vi "Control LV PowerSupply.vi"(8 "error in":errorcluster, 9 "Socket Index":i16, 11 "PPS Config In":T1={"VISA Resource"="", "Voltage Level (0.0 V)"=0.0, "CURRent Limit (0.0 A)"=0.0, "OVP LEVEL (0V)"=0.0, "Enable OVP (T: Enable)"=TRUE, "OCP LEVEL (0A)"=0.0, "Enable OCP (T: Enable)"=TRUE, "Value Out"="", "Value In"="", "Actual Voltage Level (V)"=0.0, "Actual Current Limit (A)"=0.0, "Select Instrument"="", "Enable Output"=FALSE, "PPS Operation"=enum."Close", "Type"=0} {"Type" items=["Voltage", "Current"]; "Actual Current Limit (A)" format="%.2f"; "Actual Voltage Level (V)" format="%.2f"; "OCP LEVEL (0A)" format="%.2f"; "OVP LEVEL (0V)" format="%.2f"; "Voltage Level (0.0 V)" format="%.2f"}) -> (0 "error out":errorcluster, 2 "Report Text":string, 3 "PPS Config Out":T1={"VISA Resource"="", "Voltage Level (0.0 V)"=0.0, "CURRent Limit (0.0 A)"=0.0, "OVP LEVEL (0V)"=0.0, "Enable OVP (T: Enable)"=TRUE, "OCP LEVEL (0A)"=0.0, "Enable OCP (T: Enable)"=TRUE, "Value Out"="", "Value In"="", "Actual Voltage Level (V)"=0.0, "Actual Current Limit (A)"=0.0, "Select Instrument"="", "Enable Output"=FALSE, "PPS Operation"=enum."Close", "Type"=0} {"Type" items=["Voltage", "Current"]; "Actual Current Limit (A)" format="%.2f"; "Actual Voltage Level (V)" format="%.2f"; "OCP LEVEL (0A)" format="%.2f"; "OVP LEVEL (0V)" format="%.2f"; "Voltage Level (0.0 V)" format="%.2f"})   [LabVIEW 2023, in "HardwareAbstractionLayer_LVOOP.lvlib" / "Wait Monitor.lvclass"]
uses:
  Wait Monitor.lvclass
  PowerSupply/Teststand/Control/PPS StepType Control.ctl
  PowerSupply/IT-M3904D/IT-M3904D.lvclass
  PowerSupply/Control/PPS Configure Data.ctl
  PowerSupply/PowerSupply.lvclass
  Database/Database.lvclass
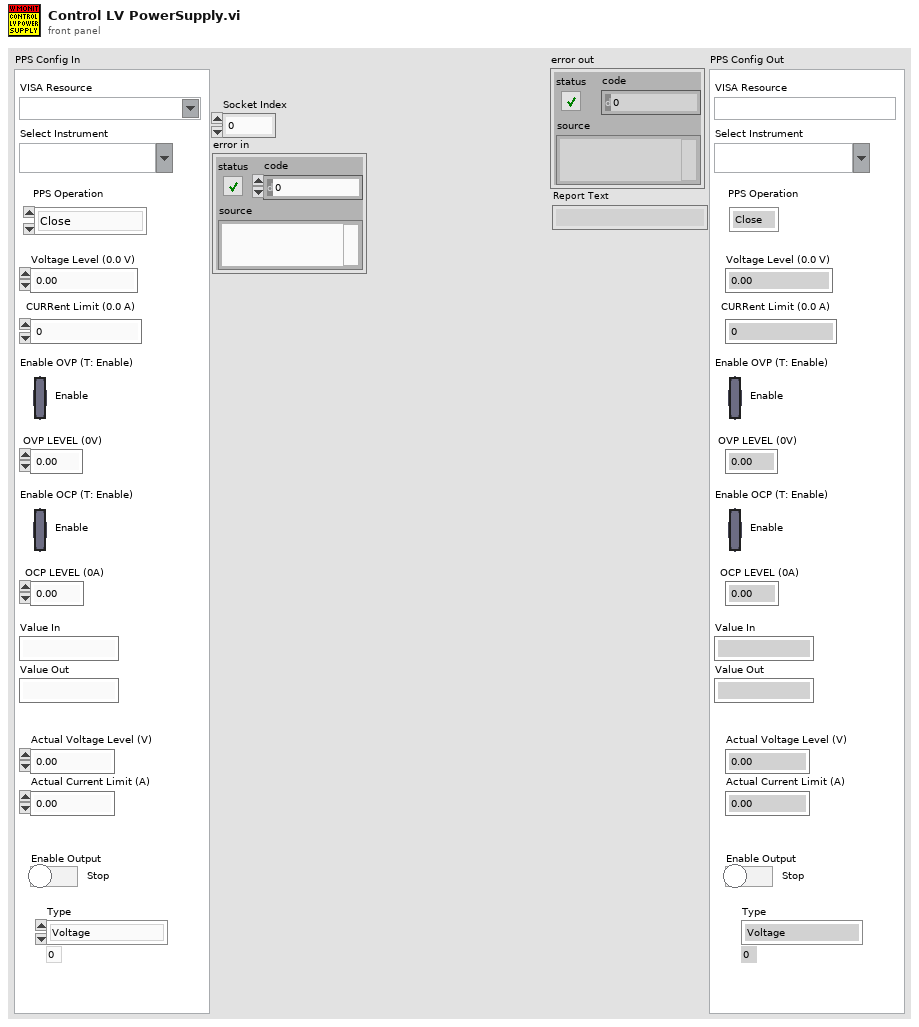
[diagram p1: front panel]
types:
  T1 = typedef "HardwareAbstractionLayer_LVOOP.lvlib/PowerSupply.lvclass/PPS StepType Control.ctl" = cluster{"VISA Resource":refnum<visa-resource-name>, "Voltage Level (0.0 V)":dbl, "CURRent Limit (0.0 A)":dbl, "OVP LEVEL (0V)":dbl, "Enable OVP (T: Enable)":bool, "OCP LEVEL (0A)":dbl, "Enable OCP (T: Enable)":bool, "Value Out":string, "Value In":string, "Actual Voltage Level (V)":dbl, "Actual Current Limit (A)":dbl, "Select Instrument":string, "Enable Output":bool, "PPS Operation":enum32{"Init", "Self Test", "Configure", "Measure", "Close"}, "Type":u16}
  T2 = typedef "HardwareAbstractionLayer_LVOOP.lvlib/PowerSupply.lvclass/PPS Configure Data.ctl" = cluster{"Voltage Level (0.0 V)":dbl, "CURRent Limit (0.0 A)":dbl, "OVP LEVEL (0V)":dbl, "OCP LEVEL (0A)":dbl, "Enable OVP (T: Enable)":bool, "Enable OCP (T: Enable)":bool, "Enable Output ":bool, "Delays OCP":dbl, "Delays OVP":dbl, "Mode(0:Voltage)":u16, "CURRent Level (0.0 A)":dbl, "Voltage Limit (0.0 V)":dbl}
  T3 = enum32{"Init", "Self Test", "Configure", "Measure", "Close"}
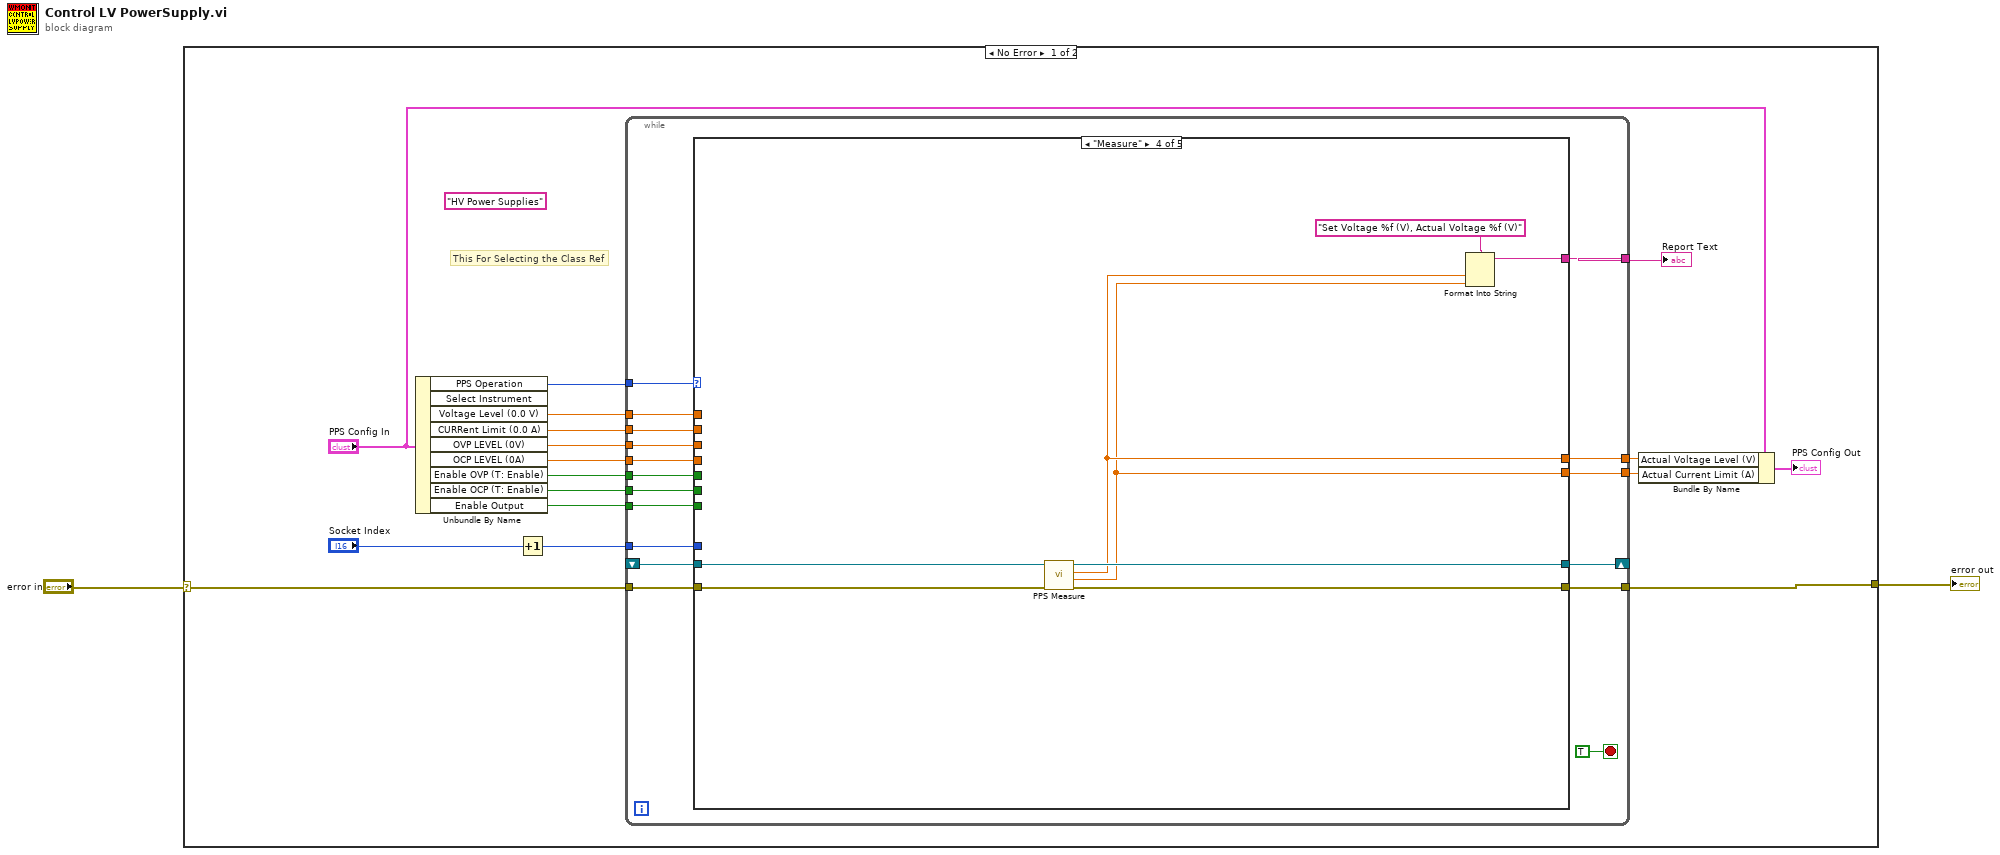
[diagram p0: block diagram]
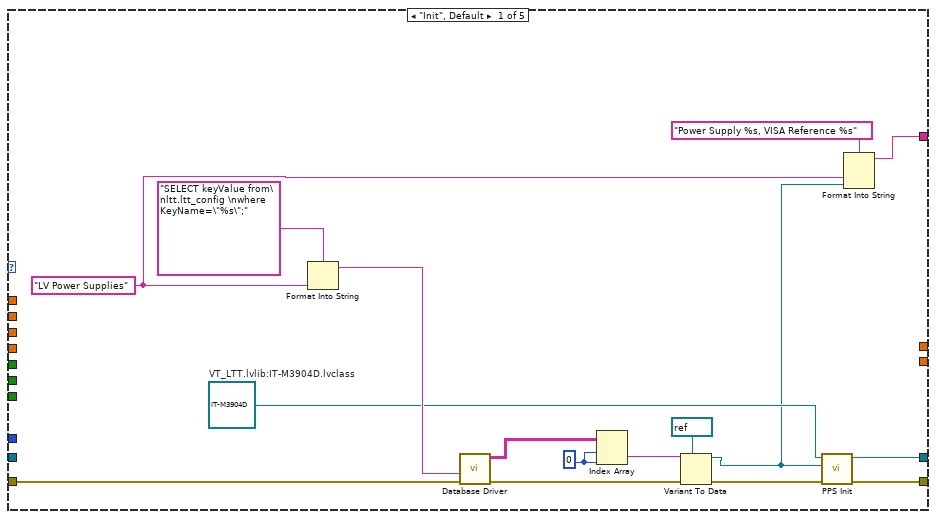
[diagram p2: hidden frame]
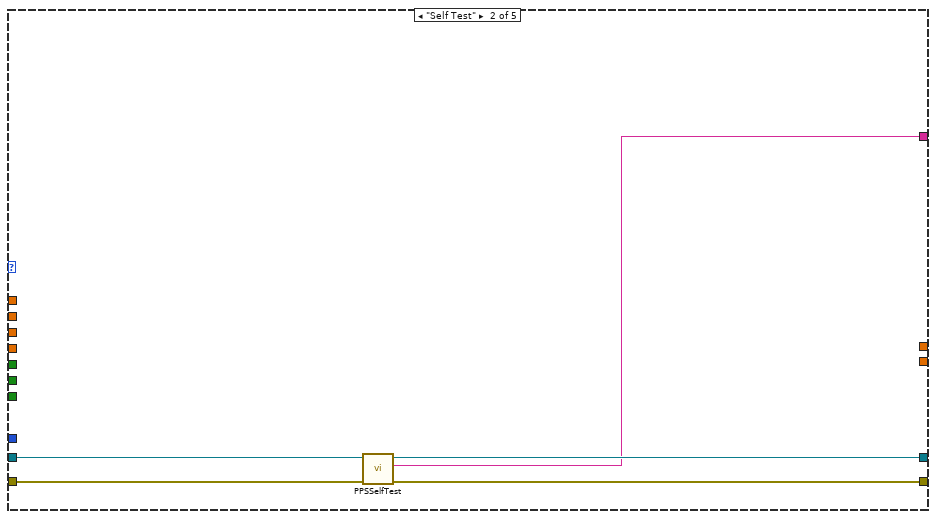
[diagram p3: hidden frame]
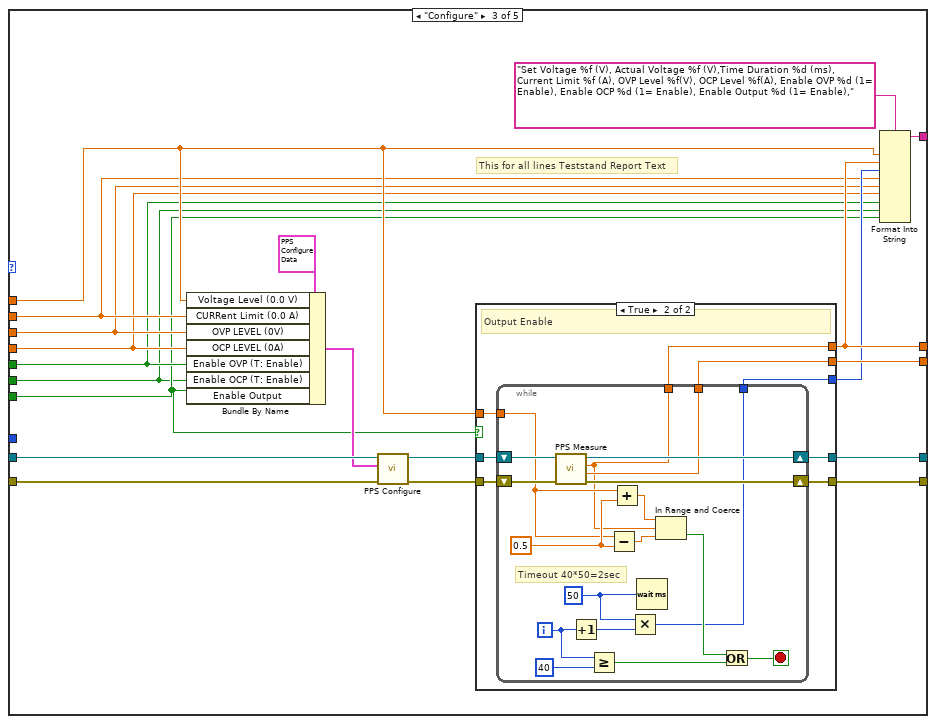
[diagram p4: hidden frame]
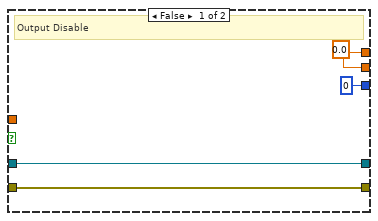
[diagram p5: hidden frame]
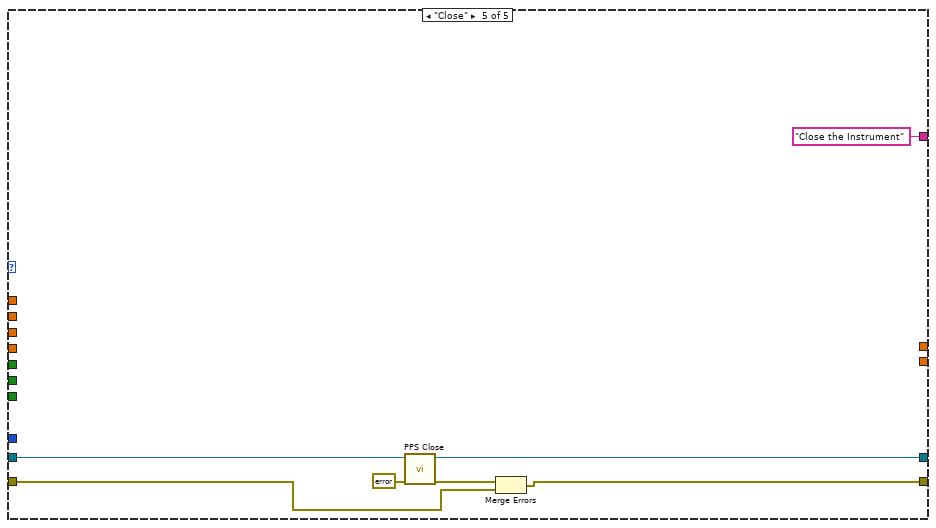
[diagram p6: hidden frame]
diagram:
  n1 = case shown="No Error" "error in" {
    selector: "error in" -> [w18 w123]
    tunnel: [w17 w123] -> w1
    frame No Error {
      (unwired) "HV Power Supplies" ("Select Instrument")
      # "This For Selecting the Class Ref"
      n2 = Unbundle By Name("PPS Config In") -> ("PPS Operation"=w19:T3, "Voltage Level (0.0 V)"=w16:dbl, "CURRent Limit (0.0 A)"=w15:dbl, "OVP LEVEL (0V)"=w14:dbl, "OCP LEVEL (0A)"=w13:dbl, "Enable OVP (T: Enable)"=w12:bool, "Enable OCP (T: Enable)"=w11:bool, "Enable Output"=w10:bool)  [unwired: 1 out]
      n3 = Increment(x="Socket Index") -> (x+1=w3:i16)
      n4 = while {
        tunnel: w19 -> [w35]
        shift-right: [w32] -> _
        shift-left: _ -> [w31]
        tunnel: w16 -> [w30]
        tunnel: w15 -> [w29]
        tunnel: w14 -> [w28]
        tunnel: w13 -> [w27]
        tunnel: w12 -> [w26]
        tunnel: w11 -> [w25]
        tunnel: w10 -> [w24]
        tunnel: w3 -> [w23]
        tunnel: [w22] -> w8
        tunnel: [w21] -> w5
        tunnel: [w20] -> w4
        tunnel: w18 -> [w34]
        tunnel: [w33] -> w17
        stop <- TRUE stop-if-true
        n5 = case shown="\"Measure\"" w35 {
          tunnel: w34 -> [w44 w56 w76 w114 w116]
          tunnel: [w52 w55 w73 w113 w117] -> w33
          tunnel: [w51 w54 w72 w112 w120] -> w32
          tunnel: w31 -> [_ w57 w77 w115 w121]
          tunnel: w30 -> [_ _ w69 _ _]
          tunnel: w29 -> [_ _ w63 _ _]
          tunnel: w28 -> [_ _ w62 _ _]
          tunnel: w27 -> [_ _ w61 _ _]
          tunnel: w26 -> [_ _ w60 _ _]
          tunnel: w25 -> [_ _ w58 _ _]
          tunnel: w24 -> [_ _ w59 _ _]
          tunnel: w23 -> [_ _ _ _ _]
          tunnel: [w41 w53 w68 w110 "Close the Instrument" ("Self-Test Result Message")] -> w22
          tunnel: [_ _ w67 w109 _] -> w21
          tunnel: [_ _ w66 w108 _] -> w20
          frame "Init", Default {
            w37 = "LV Power Supplies" ("input 1")
            w42 = refnum<class "IT-M3904D.lvclass"> refnum  # VT_LTT.lvlib:IT-M3904D.lvclass
            w50 = 0 ("index (row)")
            n6 = Format Into String(format string="SELECT keyValue from\nltt.ltt_config \nwhere KeyName=\"%s\";", w37) -> (resulting string=w46:string)  [unwired: 2 in, 1 out]
            n7 = call "Database Driver.vi"("error in"=w44, "SQL query"=w46) -> ("error out"=w43:errorcluster, "data"=w45:string[][])  [unwired: 6 in, 2 out]
            n8 = Index Array(array=w45, index (row)=w50, index (col)=w50) -> (element=w47:string)
            n9 = Variant To Data(error in=w43, type=refnum<visa-resource-name> "LV" ("VISA resource name"), Variant=w47) -> (data=w39:refnum<visa-resource-name>, error out=w49:errorcluster)
            n10 = call-dynamic "PPS Init.vi"("error in (no error)"=w49, "VISA resource name"=w39, "IT-M3904D in"=w42) -> ("error out"=w52:errorcluster, "IT-M3904D out"=w51:refnum<class "IT-M3904D.lvclass">)  [unwired: 7 in]
            n11 = Format Into String(format string="Power Supply %s, VISA Reference %s", w37, w39) -> (resulting string=w41:string)  [unwired: 2 in, 1 out]
          }
          frame "Self Test" {
            n12 = call-dynamic "PPSSelfTest.vi"("error in (no error)"=w56, "PowerSupply in"=w57) -> ("error out"=w55:errorcluster, "Self-Test Result Message"=w53:string, "PowerSupply out"=w54:refnum<class "PowerSupply.lvclass">)  [unwired: 7 in]
          }
          frame "Configure" {
            # "This for all lines Teststand Report Text"
            n13 = Bundle By Name(cluster=T2 {"Voltage Level (0.0 V)"=0.0, "CURRent Limit (0.0 A)"=0.0, "OVP LEVEL (0V)"=0.0, "OCP LEVEL (0A)"=0.0, "Enable OVP (T: Enable)"=TRUE, "Enable OCP (T: Enable)"=TRUE, "Enable Output "=TRUE, "Delays OCP"=0.0, "Delays OVP"=0.0, "Mode(0:Voltage)"=0, "CURRent Level (0.0 A)"=0.0, "Voltage Limit (0.0 V)"=0.0} ("Configure"), "Voltage Level (0.0 V)"=w69, "CURRent Limit (0.0 A)"=w63, "OVP LEVEL (0V)"=w62, "OCP LEVEL (0A)"=w61, "Enable OVP (T: Enable)"=w60, "Enable OCP (T: Enable)"=w58, "Enable Output"=w59) -> (w74:T2)
            n14 = call-dynamic "PPS Configure.vi"("error in (no error)"=w76, "Configure"=w74, "PowerSupply in"=w77) -> ("error out"=w65:errorcluster, "PowerSupply out"=w71:refnum<class "PowerSupply.lvclass">)  [unwired: 7 in]
            n15 = case shown="True" w59 {
              tunnel: w65 -> [w80 w89]
              tunnel: [w80 w88] -> w73
              tunnel: [w81 w87] -> w72
              tunnel: w71 -> [w81 w86]
              tunnel: w69 -> [_ w83]
              tunnel: [w79 w85] -> w67
              tunnel: [w79 w84] -> w66
              tunnel: [u32 0 w82] -> w64
              frame False {
                w79 = 0.0 ("Actual Voltage Level (V)")
                # "Output Disable"
              }
              frame True {
                # "Output Enable"
                n16 = while {
                  tunnel: [w95] -> w85
                  tunnel: [w103] -> w84
                  shift-right: [w106] -> w88
                  shift-left: w89 -> [w107]
                  shift-right: [w105] -> w87
                  shift-left: w86 -> [w104]
                  tunnel: w83 -> [w96]
                  tunnel: [w93] -> w82
                  i -> [w92]
                  stop <- w100 stop-if-true
                  w98 = 0.5
                  w94 = u32 50 ("milliseconds to wait")
                  # "Timeout 40*50=2sec"
                  n17 = call-dynamic "PPS Measure.vi"("error in (no error)"=w107, "PowerSupply in"=w104) -> ("error out"=w106:errorcluster, "Actual Current Limit (A)"=w103:dbl, "Actual Voltage Level (V)"=w95:dbl, "PowerSupply out"=w105:refnum<class "PowerSupply.lvclass">)  [unwired: 6 in]
                  n18 = Increment(x=w92) -> (x+1=w90:i32)
                  n19 = Greater Or Equal?(x=w92, y=40) -> (x >= y?=w102:bool)
                  n20 = Subtract(x=w96, y=w98) -> (x-y=w97:dbl)
                  n21 = Add(x=w96, y=w98) -> (x+y=w99:dbl)
                  n22 = Multiply(x=w94, y=w90) -> (x*y=w93:u32)
                  n23 = Wait (ms)(milliseconds to wait=w94) -> ()  [unwired: 1 out]
                  n24 = In Range and Coerce(upper limit=w99, x=w95, lower limit=w97) -> (In Range?=w101:bool)  [unwired: 1 out]
                  n25 = Or(x=w101, y=w102) -> (x .or. y?=w100:bool)
                }
              }
            }
            n26 = Format Into String(format string="Set Voltage %f (V), Actual Voltage %f (V),Time Duration %d (ms), Current Limit %f (A), OVP Level %f(V), OCP Level %f(A), Enable OVP %d (1= Enable), Enable OCP %d (1= Enable), Enable Output %d (1= Enable),", w69, w67, w64, w63, w62, w61, w60, w58, w59) -> (resulting string=w68:string)  [unwired: 2 in, 1 out]
          }
          frame "Measure" {
            n27 = call-dynamic "PPS Measure.vi"("error in (no error)"=w114, "PowerSupply in"=w115) -> ("error out"=w113:errorcluster, "Actual Current Limit (A)"=w108:dbl, "Actual Voltage Level (V)"=w109:dbl, "PowerSupply out"=w112:refnum<class "PowerSupply.lvclass">)  [unwired: 6 in]
            n28 = Format Into String(format string="Set Voltage %f (V), Actual Voltage %f (V)", w109, w108) -> (resulting string=w110:string)  [unwired: 2 in, 1 out]
          }
          frame "Close" {
            n29 = call-dynamic "PPS Close.vi"("error in (no error)"=errorcluster {"status"=FALSE, "code"=0, "source"=""}, "PowerSupply in"=w121) -> ("error out"=w122:errorcluster, "PowerSupply out"=w120:refnum<class "PowerSupply.lvclass">)  [unwired: 8 in]
            n30 = Merge Errors(w122, w116) -> (w117:errorcluster)
          }
        }
      }
      "Report Text" <- w8
      n31 = Bundle By Name(cluster="PPS Config In", "Actual Voltage Level (V)"=w5, "Actual Current Limit (A)"=w4) -> (→"PPS Config Out":T1)
    }
    frame Error {
    }
  }
  "error out" <- w1
